vi "DoesPathInvolveTackTest.vi"() -> (3 "Were there any errors at all?":bool)   [LabVIEW 2013]
uses:
  Data/TypeDefs/Sailing Regimes.ctl
panel:
  in  "Suggested regime modification":i32[](array[numeric])=[-1, -1, 1, 1, 1, -1, 1, -1]
  in  "Desired regime inputs":T1[](array[typedef])=[enum."Reach - Starboard Tack", enum."Run - Starboard Tack", enum."Reach - Port Tack", enum."Upwind - Port Tack", enum."Upwind - Starboard Tack", enum."Upwind - Port Tack", enum."Reach - Starboard Tack", enum."Reach - Starboard Tack"]
  out "Actual output booleans":bool[](array[boolean])
  in  "Expected output booleans":bool[](array[boolean])=[FALSE, TRUE, TRUE, FALSE, TRUE, TRUE, TRUE, FALSE]
  in  "Current regime inputs":T1[](array[typedef])=[enum."Run - Starboard Tack", enum."Reach - Starboard Tack", enum."Upwind - Port Tack", enum."Reach - Port Tack", enum."Upwind - Port Tack", enum."Upwind - Starboard Tack", enum."Run - Port Tack", enum."Run - Port Tack"]
  out "Are chosen regimes right?":bool[](array[boolean])=[TRUE, TRUE, TRUE, TRUE, TRUE, TRUE]
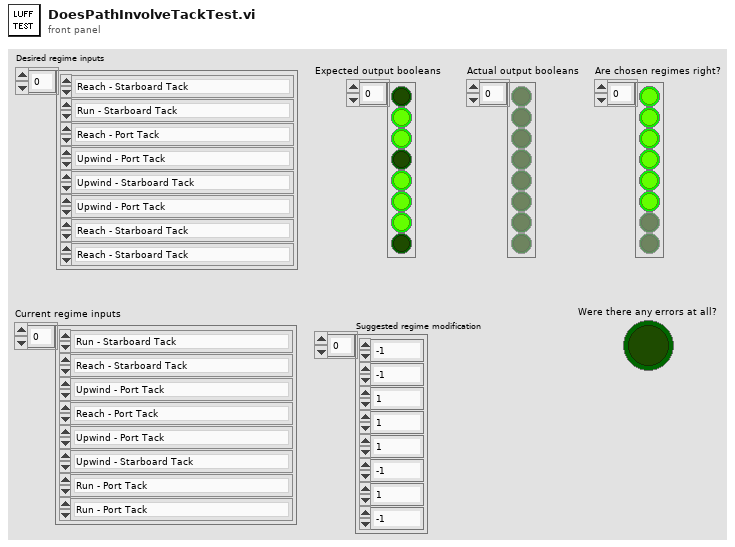
[diagram p1: front panel]
types:
  T1 = typedef "Sailing Regimes.ctl" = enum16{"Tack - Bow across wind", "Upwind - Starboard Tack", "Turn between Upwind/Reach - Starboard Tack", "Reach - Starboard Tack", "Turn between Reach/Run - Starboard Tack", "Run - Starboard Tack", "Jibe - Stern across wind", "Run - Port Tack", "Turn between Reach/Run - Port Tack", "Reach - Port Tack", "Turn between Upwind/Reach - Port Tack", "Upwind - Port Tack"}
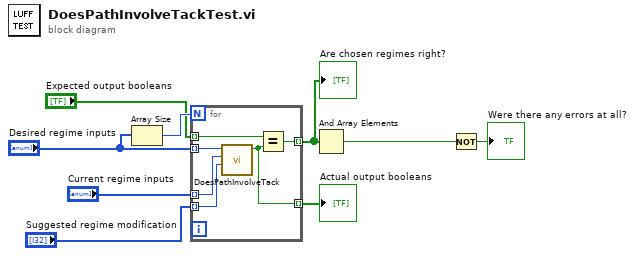
[diagram p0: block diagram]
diagram:
  n1 = Array Size(array="Desired regime inputs") -> (size(s)=w9:i32)
  n2 = for {
    N: w9 -> [_]
    tunnel: "Expected output booleans" -> [w15] mode=indexing
    tunnel: [w14] -> w8 mode=indexing
    tunnel: "Current regime inputs" -> [w12] mode=indexing
    tunnel: [w13] -> w3 mode=indexing
    tunnel: "Desired regime inputs" -> [w11] mode=indexing
    tunnel: "Suggested regime modification" -> [w10] mode=indexing
    n3 = call "DoesPathInvolveTack.vi"("Suggested regime modification"=w10, "Current Sailing Regime"=w12, "Desired Sailing Regime"=w11) -> ("Path involves tack?"=w13:bool)  [unwired: 8 in]
    n4 = Equal?(x=w15, y=w13) -> (x = y?=w14:bool)
  }
  "Are chosen regimes right?" <- w8
  "Actual output booleans" <- w3
  n5 = And Array Elements(Boolean array=w8) -> (logical AND=w6:bool)
  n6 = Not(x=w6) -> (.not. x?=→"Were there any errors at all?":bool)
